vi "intStringToInt.vi"(8 "Error in (no error)":errorcluster, 9 "String format (decimal)":T1=10 items=["Binary"=2, "Octal"=8, "Decimal"=10, "Hexadecimal"=16, "Hexatrigesimal"=36, "ASCII"=64], 10 "String in":string) -> (0 "Error out":errorcluster, 3 "Int out":refnum<class "IntClass.lvclass">)   [LabVIEW 2011, in "IntClass.lvclass"]
uses:
  IntClass.lvclass
  UintClass/enumBase.ctl
  IntClass.lvclass/IntClass.ctl
  UintClass/UintClass.lvclass
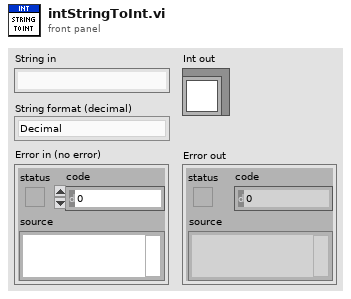
[diagram p1: front panel]
types:
  T1 = typedef "UintClass.lvclass/enumBase.ctl" = u16
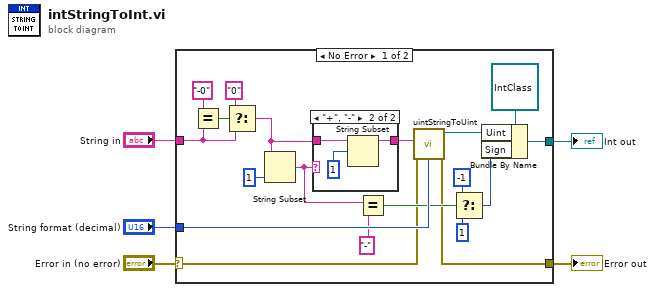
[diagram p0: block diagram]
diagram:
  n1 = case shown="No Error" "Error in (no error)" {
    selector: "Error in (no error)" -> [w12 w29]
    tunnel: [w11 w29] -> w5
    tunnel: "String in" -> [w7 _]
    tunnel: "String format (decimal)" -> [w22 _]
    tunnel: [w13 _] -> w1
    frame No Error {
      n2 = Equal?(x="-0" ("y"), y=w7) -> (x = y?=w10:bool)
      n3 = Select(t="0" ("y"), s=w10, f=w7) -> (s? t:f=w6:string)
      n4 = String Subset(string=w6, length (rest)=1 ("length (rest)")) -> (substring=w19:string)  [unwired: 1 in]
      n5 = case shown="\"+\", \"-\"" w19 {
        tunnel: w6 -> [w25 w27]
        tunnel: [w25 w26] -> w23
        frame Default {
        }
        frame "+", "-" {
          n6 = String Subset(string=w27, offset (0)=1) -> (substring=w26:string)  [unwired: 1 in]
        }
      }
      n7 = Equal?(x=w19, y="-") -> (x = y?=w17:bool)
      n8 = call "uintStringToUint.vi"("Error in (no error)"=w12, "String format (decimal)"=w22, "String in"=w23) -> ("Error out"=w11:errorcluster, "Uint out"=w20:refnum<class "UintClass.lvclass">)  [unwired: 7 in]
      n9 = Select(t=i8 -1 ("length (rest)"), s=w17, f=i8 1 ("length (rest)")) -> (s? t:f=w14:i8)
      n10 = Bundle By Name(cluster=refnum<class "IntClass.lvclass"> refnum ("IntClass in"), "Uint"=w20, "Sign"=w14) -> (w13:refnum<class "IntClass.lvclass">)
    }
    frame Error {
    }
  }
  "Int out" <- w1
  "Error out" <- w5
